vi "read barcode formats.vi"(8 "error in":errorcluster, 11 "configuration file path":path) -> (0 "error out":errorcluster, 3 "Frame Barcode Formats":T1[](array[typedef]))   [LabVIEW 2018]
uses:
  05.UserVI's/BarCode/typedefs/barcode format params.ctl
  05.UserVI's/BarCode/typedefs/barcode printer types.ctl
  <vilib>/Utility/config.llb/Read Key (String).vi
  <vilib>/Utility/config.llb/Read Key (U32).vi
  <vilib>/Utility/config.llb/NI_LVConfig.lvlib
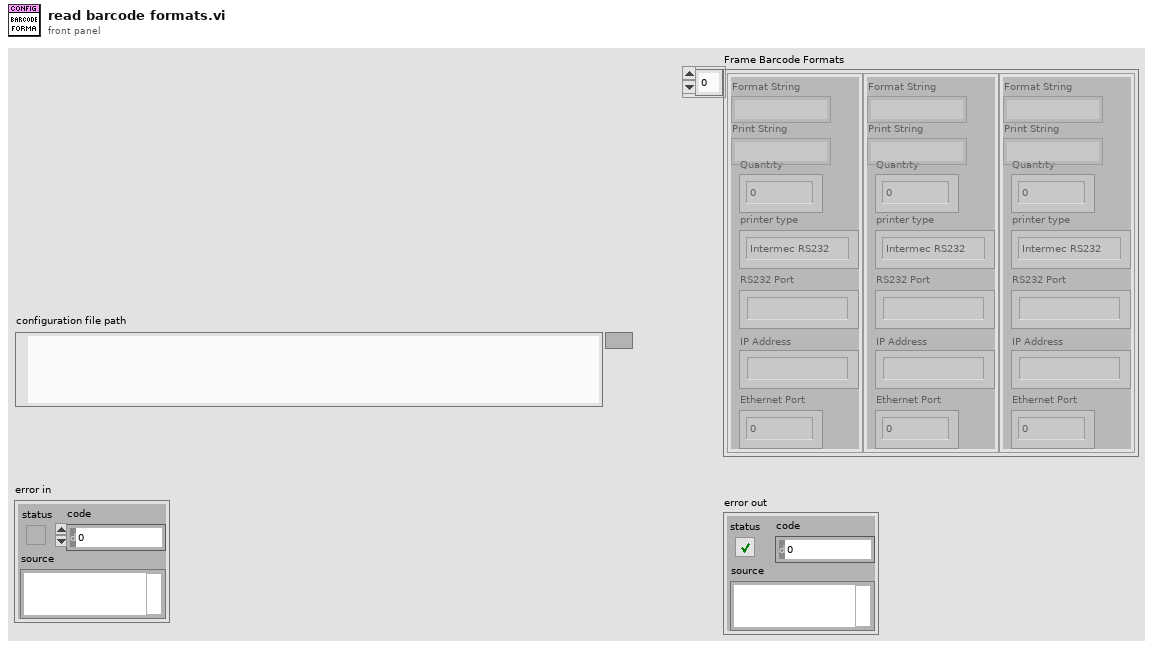
[diagram p1: front panel]
types:
  T1 = typedef "barcode format params.ctl" = cluster{"Format String":string, "Print String":string, "Quantity":u8, "printer type":T2, "RS232 Port":string, "IP Address":string, "Ethernet Port":u32}
  T2 = typedef "barcode printer types.ctl" = enum16{"Intermec RS232", "Intermec Ethernet"}
  T3 = typedef "NI_LVConfig.lvlib/Config Data RefNum.ctl" = refnum<k1>
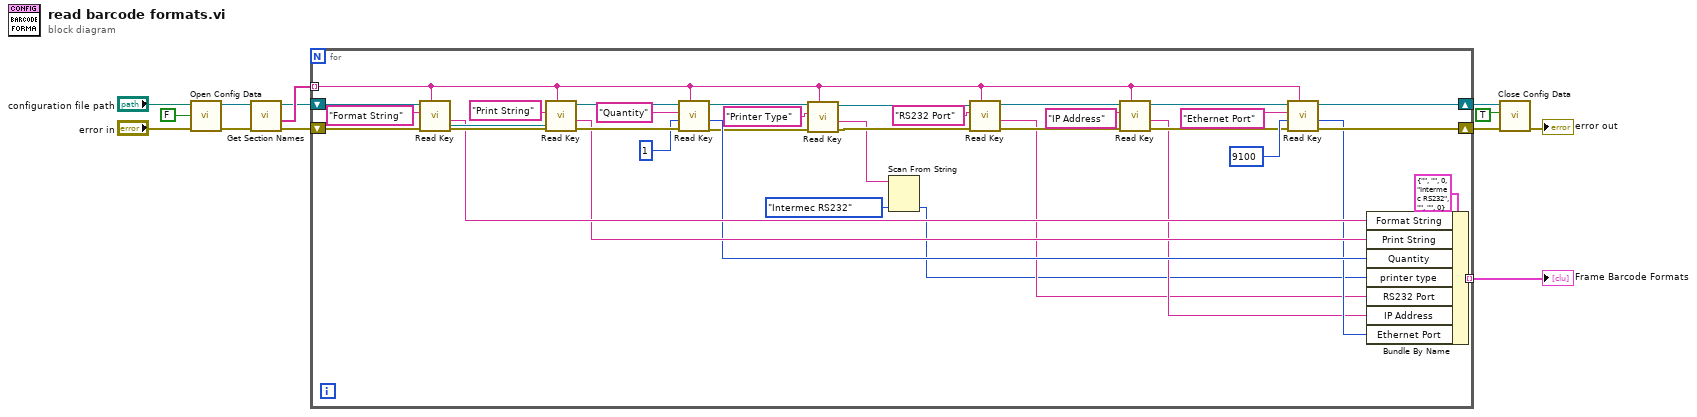
[diagram p0: block diagram]
diagram:
  n1 = call <vilib>:"Open Config Data.vi"("error in (no error)"="error in", "create file if necessary (T)"=FALSE, "configuration file path"="configuration file path") -> ("error out"=w11:errorcluster, "refnum"=w10:T3)  [unwired: 6 in, 1 out]
  n2 = call <vilib>:"Get Section Names.vi"("error in (no error)"=w11, "refnum"=w10) -> ("error out"=w6:errorcluster, "section names"=w8:string[], "refnum out"=w7:T3)  [unwired: 7 in]
  n3 = for {
    tunnel: w8 -> [w21] mode=indexing
    shift-right: [w28] -> w2
    shift-left: w7 -> [w49]
    shift-right: [w29] -> w4
    shift-left: w6 -> [w46]
    tunnel: [w37] -> w1 mode=indexing
    n4 = call-poly <vilib>:"Read Key.vi"("section"=w21, "error in (no error)"=w46, "key"="Format String", "refnum"=w49) -> ("error out"=w45:errorcluster, "value"=w40:string, "refnum out"=w48:T3)  [unwired: 2 in, 3 out]
    n5 = call-poly <vilib>:"Read Key.vi"("section"=w21, "error in (no error)"=w45, "key"="Print String", "refnum"=w48) -> ("error out"=w44:errorcluster, "value"=w39:string, "refnum out"=w43:T3)  [unwired: 2 in, 3 out]
    n6 = call-poly <vilib>:"Read Key.vi"("section"=w21, "error in (no error)"=w44, "default value"=u8 1 ("Quantity"), "key"="Quantity", "refnum"=w43) -> ("error out"=w19:errorcluster, "value"=w38:u32, "refnum out"=w20:T3)  [unwired: 1 in, 3 out]
    n7 = call-poly <vilib>:"Read Key.vi"("section"=w21, "error in (no error)"=w19, "key"="Printer Type", "refnum"=w20) -> ("error out"=w17:errorcluster, "value"=w16:string, "refnum out"=w18:T3)  [unwired: 2 in, 3 out]
    n8 = Scan From String(input string=w16, default 1=barcode_printer_types."Intermec RS232" ("printer type")) -> (output 1=w14:T2)  [unwired: 3 in, 3 out]
    n9 = call-poly <vilib>:"Read Key.vi"("section"=w21, "error in (no error)"=w17, "key"="RS232 Port", "refnum"=w18) -> ("error out"=w31:errorcluster, "value"=w23:string, "refnum out"=w26:T3)  [unwired: 2 in, 3 out]
    n10 = call-poly <vilib>:"Read Key.vi"("section"=w21, "error in (no error)"=w31, "key"="IP Address", "refnum"=w26) -> ("error out"=w30:errorcluster, "value"=w24:string, "refnum out"=w27:T3)  [unwired: 2 in, 3 out]
    n11 = call-poly <vilib>:"Read Key.vi"("section"=w21, "error in (no error)"=w30, "default value"=u32 9100 ("Quantity"), "key"="Ethernet Port", "refnum"=w27) -> ("error out"=w29:errorcluster, "value"=w25:u32, "refnum out"=w28:T3)  [unwired: 1 in, 3 out]
    n12 = Bundle By Name(cluster=T1 {"Format String"="", "Print String"="", "Quantity"=0, "printer type"=enum."Intermec RS232", "RS232 Port"="", "IP Address"="", "Ethernet Port"=0}, "Format String"=w40, "Print String"=w39, "Quantity"=w38, "printer type"=w14, "RS232 Port"=w23, "IP Address"=w24, "Ethernet Port"=w25) -> (w37:T1)
  }
  "Frame Barcode Formats" <- w1
  n13 = call <vilib>:"Close Config Data.vi"("error in (no error)"=w4, "write file if changed (T)"=TRUE, "refnum"=w2) -> ("error out"=→"error out":errorcluster)  [unwired: 7 in, 1 out]
